vi "TEST_bench_z_disengage_detect_der.vi"() -> ()   [LabVIEW 2017]
panel:
  out "Array":i32[](array[numeric])
  in  "Array 2":fxp<+/-,32,16>[](array[numeric])
  in  "Numeric 2":i32
  out "z_has_disengaged":bool
  out "Numeric":i32
  in  "NN":i16=4
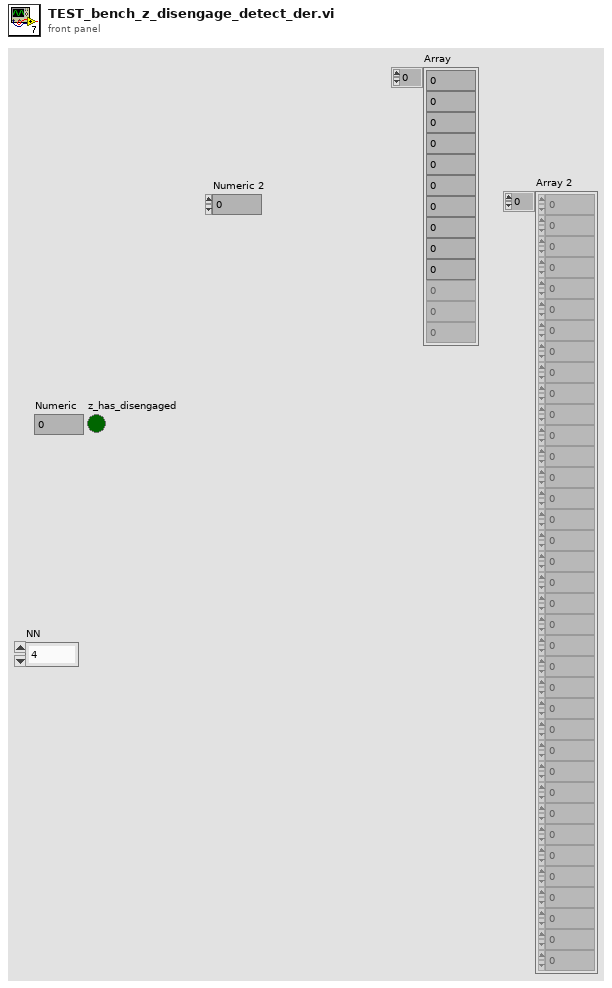
[diagram p1: front panel]
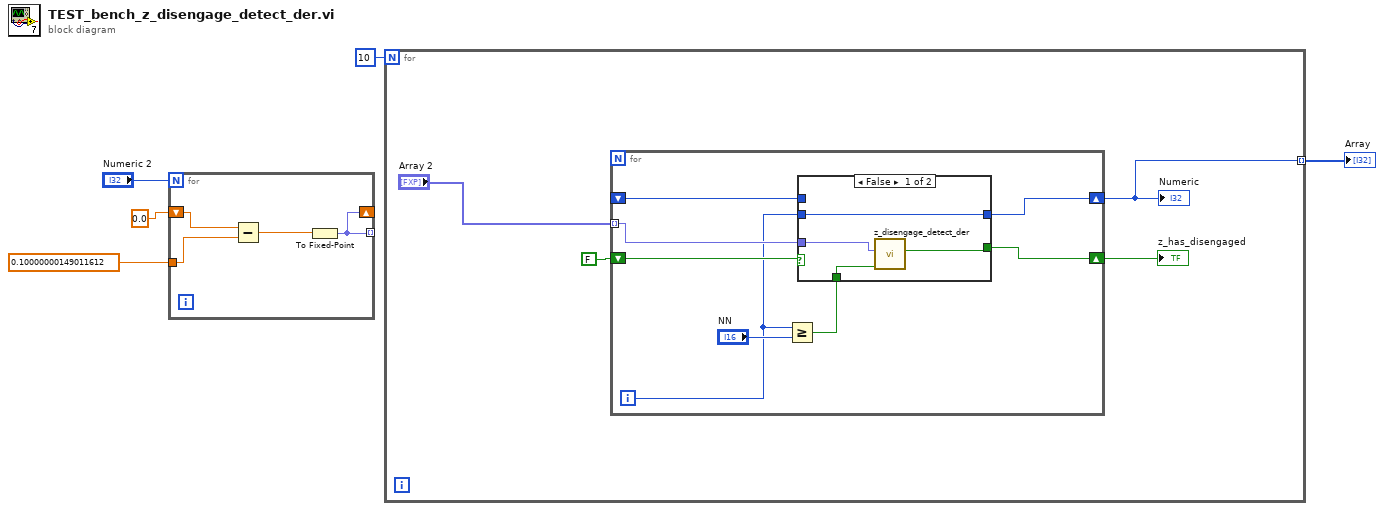
[diagram p0: block diagram]
diagram:
  n1 = for {
    N: "Numeric 2" -> [_]
    tunnel: sgl 0.1 -> [w9]
    tunnel: [w7] -> _ mode=indexing
    shift-right: [w7] -> _
    shift-left: sgl 0.0 -> [w6]
    n2 = Subtract(x=w6, y=w9) -> (x-y=w8:sgl)
    n3 = To Fixed-Point(number=w8) -> (fixed-point=w7:fxp<+/-,32,16>)  [unwired: 1 in]
  }
  n4 = for {
    N: 10 -> [_]
    tunnel: [w10] -> w1 mode=indexing
    n5 = for {
      tunnel: "Array 2" -> [w21] mode=indexing
      shift-right: [w18] -> w12
      shift-left: FALSE ("z_has_disengaged") -> [w17]
      shift-right: [w14] -> w10
      shift-left: _ -> [w15]
      i -> [w16]
      n6 = Greater Or Equal?(x=w16, y="NN") -> (x >= y?=w19:bool)
      n7 = case shown="False" w17 {
        selector: w17 -> [_ w27]
        tunnel: w21 -> [w25 _]
        tunnel: w19 -> [w23 _]
        tunnel: [w24 w27] -> w18
        tunnel: w16 -> [w22 _]
        tunnel: [w22 w26] -> w14
        tunnel: w15 -> [_ w26]
        frame False {
          n8 = call "z_disengage_detect_der.vi"("start_der_calc"=w23, "z_err"=w25) -> ("z_has_disengaged"=w24:bool)  [unwired: 9 in]
        }
        frame True {
        }
      }
    }
    "Numeric" <- w10
    "z_has_disengaged" <- w12
  }
  "Array" <- w1
